vi "3.2.0 Kalman State to Cluster.vi"(1 "State Variable X 3":T2) -> (0 "State Vector X":T1)   [LabVIEW 2011]
uses:
  <vilib>/Analysis/Matrix/Datatypes/RealMatrix.ctl
  4-High Neurons/4.2/4.2.0 Kalman State.ctl
  <vilib>/Analysis/Matrix/Numeric/Conversions/Matrix To Array - RM.vi
  <vilib>/Analysis/Matrix/NI_Matrix.lvlib
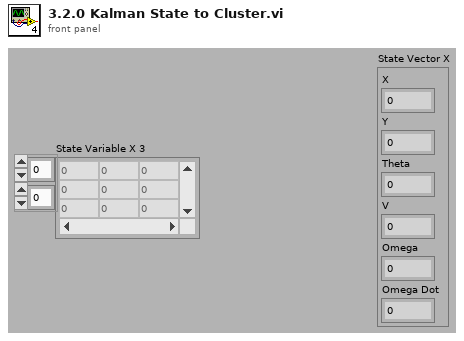
[diagram p1: front panel]
types:
  T1 = typedef "4.2.0 Kalman State.ctl" = cluster{"X":dbl, "Y":dbl, "Theta":dbl, "V":dbl, "Omega":dbl, "Omega Dot":dbl}
  T2 = typedef "NI_Matrix.lvlib/RealMatrix.ctl" = dbl[][]
  T3 = cluster{"Real 2D Array[0]":dbl, "Real 2D Array[1]":dbl, "Real 2D Array[2]":dbl, "Real 2D Array[3]":dbl, "Real 2D Array[4]":dbl, "Real 2D Array[5]":dbl}
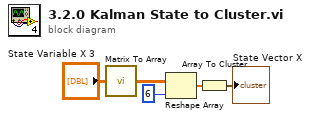
[diagram p0: block diagram]
diagram:
  n1 = call-poly <vilib>:"Matrix To Array.vi"("Real Matrix"="State Variable X 3") -> ("Real 2D Array"=w3:dbl[][])
  n2 = Reshape Array(w3, 6 ("dimension size")) -> (w5:dbl[])
  n3 = Array To Cluster(array=w5) -> (cluster=→"State Vector X":T3)
